vi "Convert Q Error to Shutdown Error.vi"(8 "error in (no error)":errorcluster) -> (0 "error out":errorcluster)   [LabVIEW 2020, in "Internal Comm Classes.lvlib" / "WPL Comm.lvclass"]
uses:
  WPL Comm.lvclass
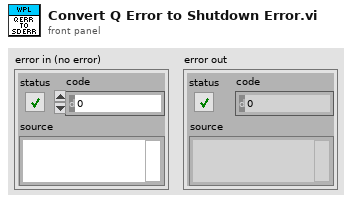
[diagram p1: front panel]
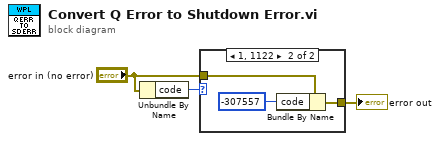
[diagram p0: block diagram]
diagram:
  n1 = Unbundle By Name("error in (no error)") -> ("code"=w3:i32)
  n2 = case shown="1, 1122" w3 {
    tunnel: [w4 w6] -> w2
    tunnel: "error in (no error)" -> [w4 w7]
    frame Default {
    }
    frame 1, 1122 {
      n3 = Bundle By Name(cluster=w7, "code"=-307557) -> (w6:errorcluster)
    }
  }
  "error out" <- w2
